vi "Construct Client Network Messenger.vi"(5 "Log Alias":string, 6 "Local Port (0)":u16, 7 "Log Instance":refnum<class "LoggerReference.lvclass">, 8 "Remote Port or Service Name":u16, 9 "Remote IP":string, 10 "Connection State Change Callback":refnum<class "IConnectionStateChangeCallback.lvclass">, 11 "Packet Return":refnum<class "IPacket Return.lvclass">) -> (0 "error out":errorcluster, 3 "Network Node":refnum<data-value>)   [LabVIEW 2020, in "Network Messenger.lvlib" / "Network Messenger.lvclass"]
uses:
  <vilib>/gpm_packages/@cs/Network-interface/Source/Network Messenger/Network Messenger.lvclass
  <vilib>/gpm_packages/@cs/Network-interface/Source/MessagingInterfaces/IConnectionStateChangeCallback/IConnectionStateChangeCallback.lvclass
  <vilib>/gpm_packages/@cs/Network-interface/Source/Network Messenger/IPacket Return/IPacket Return.lvclass
  <vilib>/gpm_packages/@cs/event-logger/Source/Composed Log/LoggerReference/LoggerReference.lvclass
  <vilib>/gpm_packages/@cs/Network-interface/Source/Network Messenger/Header Data Packet Return/Header Data Packet Return.lvclass/Header Data Packet Return.ctl
  <vilib>/gpm_packages/@cs/Network-interface/Source/Network Messenger/Write Strategy/Write Strategy.lvclass
  C:/Program Files/National Instruments/LabVIEW 2020/vi.lib/gpm_packages/@cs/Network-interface/Source/MessagingInterfaces/IWriteStrategy/IWriteStrategy.lvclass
  <vilib>/gpm_packages/@cs/Network-interface/Source/Network Messenger/ReadStrategy/ReadStrategy.lvclass
  C:/Program Files/National Instruments/LabVIEW 2020/vi.lib/gpm_packages/@cs/Network-interface/Source/MessagingInterfaces/IReadStrategy/IReadStrategy.lvclass
  <vilib>/gpm_packages/@cs/Network-interface/Source/Network Messenger/Network Messenger.lvclass/Network Messenger.ctl
  <vilib>/gpm_packages/@cs/Network-interface/Source/Create Ref Message/Create Ref Message.lvclass/Create Ref Message.ctl
  <vilib>/ActorFramework/Message Enqueuer/Message Enqueuer.lvclass/Message Enqueuer.ctl
  <vilib>/ActorFramework/Message Enqueuer/Enqueue.vi
  <vilib>/gpm_packages/@cs/Network-interface/Source/Network Messenger/Header Data Packet Return/Header Data Packet Return.lvclass
  C:/Program Files/National Instruments/LabVIEW 2020/vi.lib/gpm_packages/@cs/Network-interface/Source/MessagingInterfaces/IMessageReturnPolicy/IMessageReturnPolicy.lvclass
  <vilib>/gpm_packages/@cs/Network-interface/Source/TCP Interface/TCP Client/TCP Client.lvclass
  C:/Program Files/National Instruments/LabVIEW 2020/vi.lib/gpm_packages/@cs/Network-interface/Source/IConnectionFactory/IConnectionFactory.lvclass
  <vilib>/gpm_packages/@cs/Network-interface/Source/PersistantConnectionHandler/PersistantConnectionHandler/PersistantConnectionHandler.lvclass
  C:/Program Files/National Instruments/LabVIEW 2020/vi.lib/ActorFramework/Actor/Actor.lvclass
  <vilib>/gpm_packages/@cs/Network-interface/Source/Create Ref Message/Create Ref Message.lvclass
  C:/Program Files/National Instruments/LabVIEW 2020/vi.lib/ActorFramework/Message/Message.lvclass
  <vilib>/ActorFramework/Message Priority Queue/Priority Enqueue.vi
  <vilib>/ActorFramework/Actor/Actor.lvclass
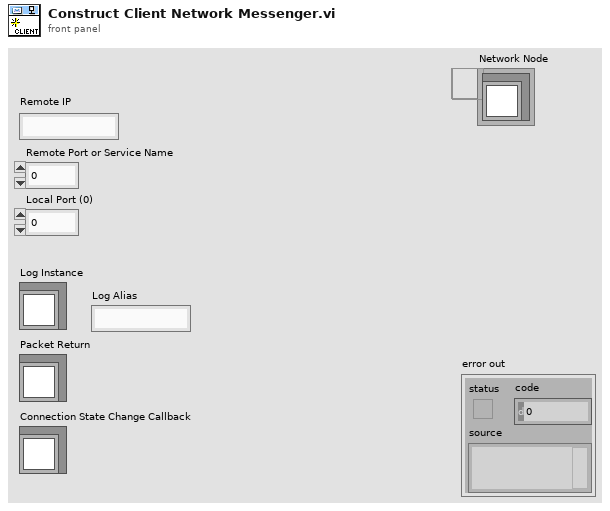
[diagram p1: front panel]
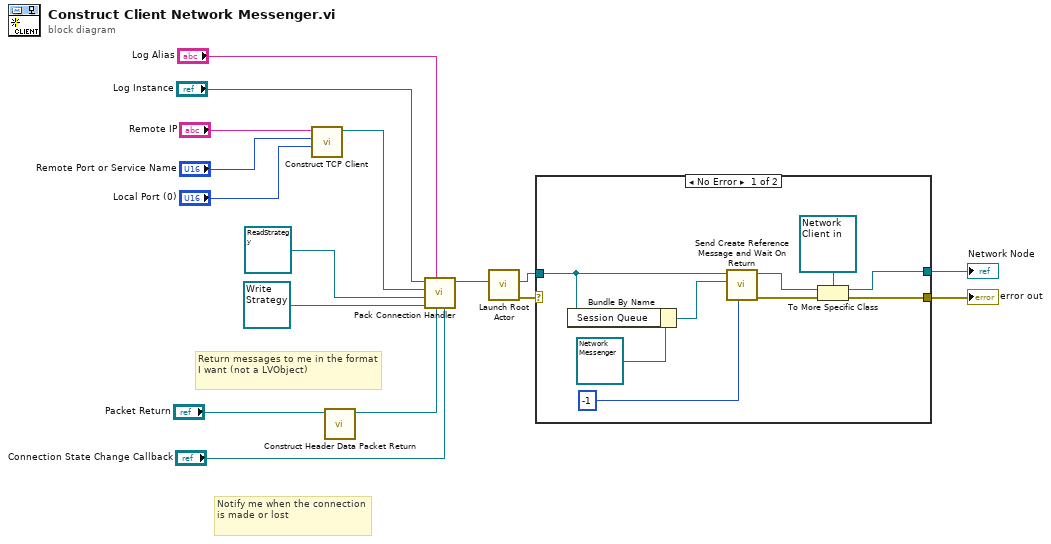
[diagram p0: block diagram]
diagram:
  # "Return messages to me in the format I want (not a LVObject)"
  # "Notify me when the connection is made or lost"
  n1 = call <vilib>:"Construct TCP Client.vi"("Local Port (0)"="Local Port (0)", "Remote Port or Service Name"="Remote Port or Service Name", "Address"="Remote IP") -> ("TCP Client out"=w12:refnum<class "TCP Client.lvclass">)  [unwired: 8 in]
  n2 = call <vilib>:"Construct Header Data Packet Return.vi"("Packet Return"="Packet Return") -> ("Header Data Packet Return out"=w11:refnum<class "Header Data Packet Return.lvclass">)  [unwired: 10 in]
  n3 = call <vilib>:"Pack Connection Handler.vi"("State Change Callback"="Connection State Change Callback", "Message Return Policy"=w11, "Log Alias"="Log Alias", "Write Strategy"=refnum<class "Write Strategy.lvclass"> refnum ("Network Messenger.lvlib:Write Strategy.lvclass"), "Read Strategy"=refnum<class "ReadStrategy.lvclass"> refnum ("Network Messenger.lvlib:ReadStrategy.lvclass"), "Connection Factory Type"=w12, "Log Instance"="Log Instance") -> ("PersistantConnectionHandler out"=w9:refnum<class "PersistantConnectionHandler.lvclass">)  [unwired: 4 in]
  n4 = call <vilib>:"Launch Root Actor.vi"("Actor"=w9) -> ("error out"=w8:errorcluster, "Actor's Enqueuer"=w7:refnum<class "Message Enqueuer.lvclass">)  [unwired: 9 in]
  n5 = case shown="No Error" w8 {
    selector: w8 -> [_ w26]
    tunnel: w7 -> [w24 _]
    tunnel: [w20 _] -> w6
    tunnel: [w19 w26] -> w5
    frame No Error {
      n6 = Bundle By Name(cluster=refnum<class "Network Messenger.lvclass"> refnum ("Network Client in"), "Session Queue"=w24) -> (w25:refnum<class "Network Messenger.lvclass">)
      n7 = call <vilib>:"Send Create Reference Message and Wait On Return.vi"("timeout in ms (-1)"=-1, "Object"=w25, "Message Enqueuer in"=w24) -> ("error out"=w23:errorcluster, "Object Reference"=w22:refnum<data-value>)  [unwired: 7 in]
      n8 = To More Specific Class(target class=refnum<data-value> refnum ("Network Node"), reference=w22, error in=w23) -> (specific class reference=w20:refnum<data-value>, error out=w19:errorcluster)
    }
    frame Error {
    }
  }
  "error out" <- w5
  "Network Node" <- w6
